vi "TCam_WellTemp.vi"(9 "Offset":dbl, 10 "Pixels":cluster{"X":i32, "Y":i32}[][](array[cluster]), 11 "Image in":T1) -> (1 "Mean Temp":dbl format="%0.2f", 2 "Image Out":T1, 3 "Temps":dbl[](array[numeric]))   [LabVIEW 2022 SP3]
uses:
  <vilib>/vision/Image Controls.llb/IMAQ Image.ctl
  <vilib>/Analysis/baseanly.llb/Mean (DBL).vi
  <vilib>/vision/NI_Vision_Development_Module.lvlib
  <vilib>/Analysis/NI_AALBase.lvlib
panel:
  out "error out":errorcluster
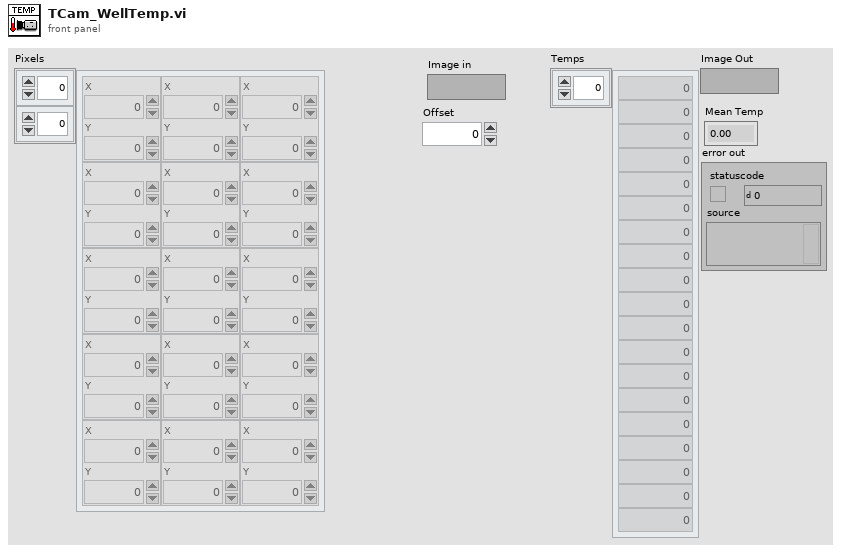
[diagram p1: front panel]
types:
  T1 = typedef "IMAQ Image.ctl" = refnum<image>
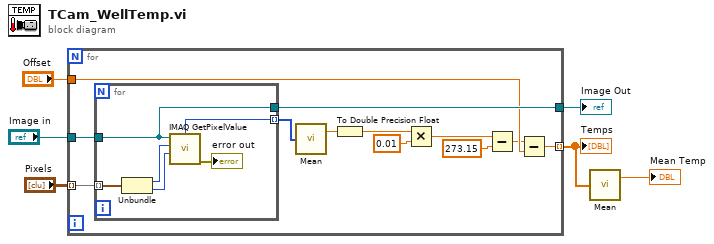
[diagram p0: block diagram]
diagram:
  n1 = for {
    tunnel: "Image in" -> [w18]
    tunnel: "Pixels" -> [w17] mode=indexing
    tunnel: [w14] -> w3 mode=indexing
    tunnel: [w15] -> w4
    tunnel: "Offset" -> [w13]
    n2 = for {
      tunnel: w18 -> [w21]
      tunnel: w17 -> [w24] mode=indexing
      tunnel: [w19] -> w16 mode=indexing
      tunnel: [w21] -> w15
      n3 = Unbundle(w24) -> ("X"=w23:i32, "Y"=w22:i32)
      n4 = call "IMAQ GetPixelValue"("Image"=w21, "X Coordinate"=w23, "Y Coordinate"=w22) -> ("Pixel Value (U16)"=w19:u16, "error out"=→"error out":errorcluster)  [unwired: 3 in, 3 out]
    }
    n5 = call-poly <vilib>:"Mean.vi"("X"=w16) -> ("mean"=w8:dbl)  [unwired: 1 out]
    n6 = To Double Precision Float(number=w8) -> (double precision float=w10:dbl)
    n7 = Multiply(x=w10, y=0.01) -> (x*y=w11:dbl)
    n8 = Subtract(x=w11, y=273.15) -> (x-y=w7:dbl)
    n9 = Subtract(x=w7, y=w13) -> (x-y=w14:dbl)
  }
  "Temps" <- w3
  "Image Out" <- w4
  n10 = call-poly <vilib>:"Mean.vi"("X"=w3) -> ("mean"=→"Mean Temp":dbl)  [unwired: 1 out]
